vi "VI Tree.vi"   [LabVIEW 2017, in "Sefram DAS220.lvlib"]
doc: "This is the instrument driver for the Sefram DAS240. The VI Tree displays all the user-callable VIs of the instrument driver in an organized table."
uses:
  <instrlib>/Sefram DAS220/Sefram DAS220.lvlib
panel:
  # "(c) 2017 Sefram Instruments.  ALL RIGHTS RESERVED."
  # "SEE DIAGRAM\nFOR VI TREE."
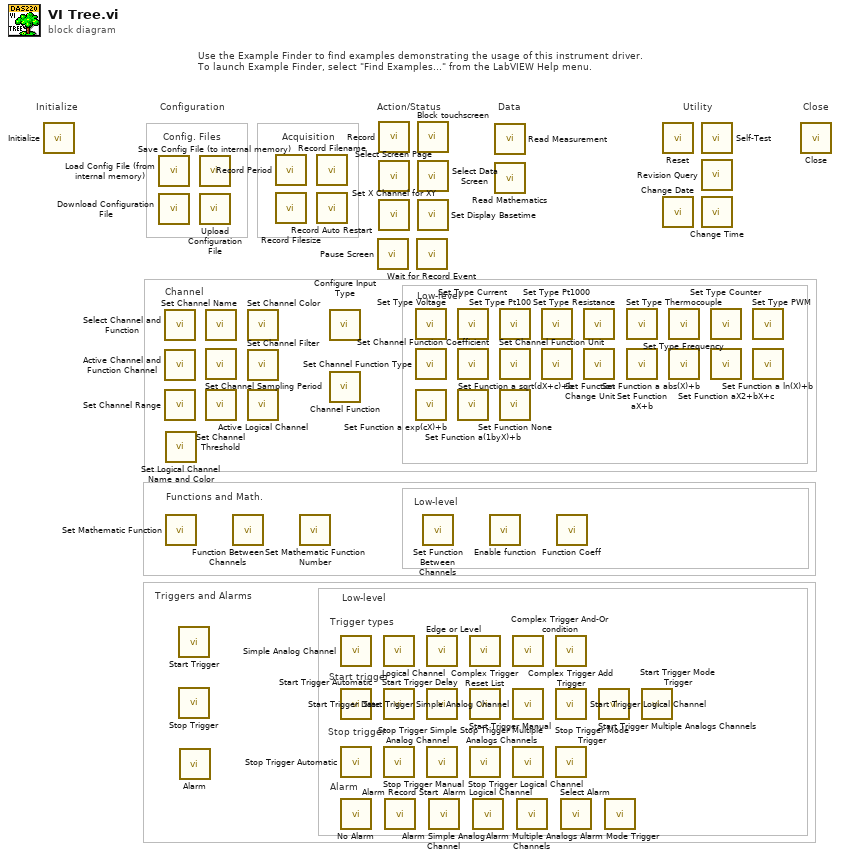
[diagram p0: block diagram]
diagram:
  # "Triggers and Alarms"
  # "Trigger types"
  # "Start trigger"
  # "Stop trigger"
  # "Alarm"
  # "Low-level"
  # "Low-level"
  # "Functions and Math."
  # "Channel"
  # "Low-level"
  # "Acquisition"
  # "Config. Files"
  # "Use the Example Finder to find examples demonstrating the usage of this instrument driver.\nTo launch Example Finder, select \"Find Examples...\" from the LabVIEW Help menu."
  # "Configuration"
  # "Utility"
  # "Data"
  # "Action/Status"
  # "Close"
  # "Initialize"
  n1 = call <instrlib>:"Initialize.vi"() -> ()  [unwired: 10 in, 2 out]
  n2 = call <instrlib>:"Load Config File (from internal memory).vi"() -> ()  [unwired: 10 in, 2 out]
  n3 = call <instrlib>:"Download Configuration File.vi"() -> ()  [unwired: 10 in, 2 out]
  n4 = call <instrlib>:"Select Channel and Function.vi"() -> ()  [unwired: 10 in, 2 out]
  n5 = call <instrlib>:"Active Channel and Function Channel.vi"() -> ()  [unwired: 10 in, 2 out]
  n6 = call <instrlib>:"Set Channel Range.vi"() -> ()  [unwired: 10 in, 2 out]
  n7 = call <instrlib>:"Set Logical Channel Name and Color.vi"() -> ()  [unwired: 10 in, 2 out]
  n8 = call <instrlib>:"Set Mathematic Function.vi"() -> ()  [unwired: 10 in, 2 out]
  n9 = call-poly <instrlib>:"Start Trigger.vi"() -> ()  [unwired: 10 in, 2 out]
  n10 = call-poly <instrlib>:"Stop Trigger.vi"() -> ()  [unwired: 10 in, 2 out]
  n11 = call-poly <instrlib>:"Alarm.vi"() -> ()  [unwired: 10 in, 2 out]
  n12 = call <instrlib>:"Save Config File (to internal memory).vi"() -> ()  [unwired: 10 in, 2 out]
  n13 = call <instrlib>:"Upload Configuration File.vi"() -> ()  [unwired: 10 in, 2 out]
  n14 = call <instrlib>:"Set Channel Name.vi"() -> ()  [unwired: 10 in, 2 out]
  n15 = call <instrlib>:"Set Channel Sampling Period.vi"() -> ()  [unwired: 10 in, 2 out]
  n16 = call <instrlib>:"Set Channel Threshold.vi"() -> ()  [unwired: 10 in, 2 out]
  n17 = call <instrlib>:"Function Between Channels.vi"() -> ()  [unwired: 18 in, 2 out]
  n18 = call <instrlib>:"Set Channel Color.vi"() -> ()  [unwired: 10 in, 2 out]
  n19 = call <instrlib>:"Set Channel Filter.vi"() -> ()  [unwired: 10 in, 2 out]
  n20 = call <instrlib>:"Active Logical Channel.vi"() -> ()  [unwired: 10 in, 2 out]
  n21 = call <instrlib>:"Record Period.vi"() -> ()  [unwired: 10 in, 2 out]
  n22 = call <instrlib>:"Record Filesize.vi"() -> ()  [unwired: 10 in, 2 out]
  n23 = call <instrlib>:"Set Mathematic Function Number.vi"() -> ()  [unwired: 10 in, 2 out]
  n24 = call <instrlib>:"Record Filename.vi"() -> ()  [unwired: 10 in, 2 out]
  n25 = call <instrlib>:"Record Auto Restart.vi"() -> ()  [unwired: 10 in, 2 out]
  n26 = call-poly <instrlib>:"Configure Input Type.vi"() -> ()  [unwired: 10 in, 2 out]
  n27 = call-poly <instrlib>:"Channel Function.vi"() -> ()  [unwired: 14 in, 2 out]
  n28 = call <instrlib>:"Simple Analog Channel.vi"() -> ()  [unwired: 10 in, 2 out]
  n29 = call <instrlib>:"Start Trigger Automatic.vi"() -> ()  [unwired: 10 in, 2 out]
  n30 = call <instrlib>:"Stop Trigger Automatic.vi"() -> ()  [unwired: 10 in, 2 out]
  n31 = call <instrlib>:"No Alarm.vi"() -> ()  [unwired: 10 in, 2 out]
  n32 = call <instrlib>:"Pause Screen.vi"() -> ()  [unwired: 10 in, 2 out]
  n33 = call <instrlib>:"Record.vi"() -> ()  [unwired: 10 in, 2 out]
  n34 = call <instrlib>:"Select Screen Page.vi"() -> ()  [unwired: 10 in, 2 out]
  n35 = call <instrlib>:"Set X Channel for XY.vi"() -> ()  [unwired: 10 in, 2 out]
  n36 = call <instrlib>:"Logical Channel.vi"() -> ()  [unwired: 10 in, 2 out]
  n37 = call <instrlib>:"Start Trigger Date.vi"() -> ()  [unwired: 10 in, 2 out]
  n38 = call <instrlib>:"Stop Trigger Manual.vi"() -> ()  [unwired: 10 in, 2 out]
  n39 = call <instrlib>:"Alarm Record Start.vi"() -> ()  [unwired: 10 in, 2 out]
  n40 = call <instrlib>:"Set Type Voltage.vi"() -> ()  [unwired: 10 in, 2 out]
  n41 = call <instrlib>:"Set Channel Function Type.vi"() -> ()  [unwired: 10 in, 2 out]
  n42 = call <instrlib>:"Set Function a exp(cX)+b.vi"() -> ()  [unwired: 14 in, 2 out]
  n43 = call <instrlib>:"Wait for Record Event.vi"() -> ()  [unwired: 10 in, 2 out]
  n44 = call <instrlib>:"Block touchscreen.vi"() -> ()  [unwired: 10 in, 2 out]
  n45 = call <instrlib>:"Select Data Screen.vi"() -> ()  [unwired: 10 in, 2 out]
  n46 = call <instrlib>:"Set Display Basetime.vi"() -> ()  [unwired: 10 in, 2 out]
  n47 = call <instrlib>:"Set Function Between Channels.vi"() -> ()  [unwired: 10 in, 2 out]
  n48 = call <instrlib>:"Edge or Level.vi"() -> ()  [unwired: 10 in, 2 out]
  n49 = call <instrlib>:"Start Trigger Delay.vi"() -> ()  [unwired: 10 in, 2 out]
  n50 = call <instrlib>:"Stop Trigger Simple Analog Channel.vi"() -> ()  [unwired: 10 in, 2 out]
  n51 = call <instrlib>:"Alarm Simple Analog Channel.vi"() -> ()  [unwired: 10 in, 2 out]
  n52 = call <instrlib>:"Set Type Current.vi"() -> ()  [unwired: 10 in, 2 out]
  n53 = call <instrlib>:"Set Channel Function Coefficient.vi"() -> ()  [unwired: 10 in, 2 out]
  n54 = call <instrlib>:"Set Function a(1byX)+b.vi"() -> ()  [unwired: 14 in, 2 out]
  n55 = call <instrlib>:"Complex Trigger Reset List.vi"() -> ()  [unwired: 10 in, 2 out]
  n56 = call <instrlib>:"Start Trigger Manual.vi"() -> ()  [unwired: 10 in, 2 out]
  n57 = call <instrlib>:"Stop Trigger Logical Channel.vi"() -> ()  [unwired: 10 in, 2 out]
  n58 = call <instrlib>:"Alarm Logical Channel.vi"() -> ()  [unwired: 10 in, 2 out]
  n59 = call <instrlib>:"Enable function.vi"() -> ()  [unwired: 10 in, 2 out]
  n60 = call <instrlib>:"Read Measurement.vi"() -> ()  [unwired: 9 in, 3 out]
  n61 = call <instrlib>:"Read Mathematics.vi"() -> ()  [unwired: 9 in, 3 out]
  n62 = call <instrlib>:"Set Type Pt100.vi"() -> ()  [unwired: 10 in, 2 out]
  n63 = call <instrlib>:"Set Channel Function Unit.vi"() -> ()  [unwired: 10 in, 2 out]
  n64 = call <instrlib>:"Set Function None.vi"() -> ()  [unwired: 14 in, 2 out]
  n65 = call <instrlib>:"Complex Trigger And-Or condition.vi"() -> ()  [unwired: 10 in, 2 out]
  n66 = call <instrlib>:"Start Trigger Simple Analog Channel.vi"() -> ()  [unwired: 10 in, 2 out]
  n67 = call <instrlib>:"Stop Trigger Multiple Analogs Channels.vi"() -> ()  [unwired: 10 in, 2 out]
  n68 = call <instrlib>:"Alarm Multiple Analogs Channels.vi"() -> ()  [unwired: 10 in, 2 out]
  n69 = call <instrlib>:"Set Type Pt1000.vi"() -> ()  [unwired: 10 in, 2 out]
  n70 = call <instrlib>:"Set Function a sqrt(dX+c)+b.vi"() -> ()  [unwired: 14 in, 2 out]
  n71 = call <instrlib>:"Complex Trigger Add Trigger.vi"() -> ()  [unwired: 10 in, 2 out]
  n72 = call <instrlib>:"Start Trigger Logical Channel.vi"() -> ()  [unwired: 10 in, 2 out]
  n73 = call <instrlib>:"Stop Trigger Mode Trigger.vi"() -> ()  [unwired: 10 in, 2 out]
  n74 = call <instrlib>:"Function Coeff.vi"() -> ()  [unwired: 10 in, 2 out]
  n75 = call <instrlib>:"Select Alarm.vi"() -> ()  [unwired: 10 in, 2 out]
  n76 = call <instrlib>:"Set Type Resistance.vi"() -> ()  [unwired: 10 in, 2 out]
  n77 = call <instrlib>:"Set Function Change Unit.vi"() -> ()  [unwired: 14 in, 2 out]
  n78 = call <instrlib>:"Start Trigger Multiple Analogs Channels.vi"() -> ()  [unwired: 10 in, 2 out]
  n79 = call <instrlib>:"Alarm Mode Trigger.vi"() -> ()  [unwired: 10 in, 2 out]
  n80 = call <instrlib>:"Set Type Thermocouple.vi"() -> ()  [unwired: 10 in, 2 out]
  n81 = call <instrlib>:"Set Function aX+b.vi"() -> ()  [unwired: 14 in, 2 out]
  n82 = call <instrlib>:"Start Trigger Mode Trigger.vi"() -> ()  [unwired: 10 in, 2 out]
  n83 = call <instrlib>:"Reset.vi"() -> ()  [unwired: 10 in, 2 out]
  n84 = call <instrlib>:"Change Date.vi"() -> ()  [unwired: 10 in, 2 out]
  n85 = call <instrlib>:"Set Type Frequency.vi"() -> ()  [unwired: 10 in, 2 out]
  n86 = call <instrlib>:"Set Function a abs(X)+b.vi"() -> ()  [unwired: 14 in, 2 out]
  n87 = call <instrlib>:"Self-Test.vi"() -> ()  [unwired: 8 in, 4 out]
  n88 = call <instrlib>:"Revision Query.vi"() -> ()  [unwired: 8 in, 4 out]
  n89 = call <instrlib>:"Change Time.vi"() -> ()  [unwired: 10 in, 2 out]
  n90 = call <instrlib>:"Set Type Counter.vi"() -> ()  [unwired: 10 in, 2 out]
  n91 = call <instrlib>:"Set Function aX2+bX+c.vi"() -> ()  [unwired: 14 in, 2 out]
  n92 = call <instrlib>:"Set Type PWM.vi"() -> ()  [unwired: 10 in, 2 out]
  n93 = call <instrlib>:"Set Function a ln(X)+b.vi"() -> ()  [unwired: 14 in, 2 out]
  n94 = call <instrlib>:"Close.vi"() -> ()  [unwired: 11 in, 1 out]
